vi "BatteryWarningTest_3.4V.vi"(8 "error in":errorcluster) -> (0 "error in (no error)":errorcluster, 1 "Pass/Fail":bool, 4 "Limit2":u8[](array[numeric]) format="%x", 5 "Limit1":u8[](array[numeric]) format="%x")   [LabVIEW 2009]
uses:
  Global/Global 1.vi
  <vilib>/Instr/_visa.llb/VISA Configure Serial Port (Instr).vi
panel:
  # "30"
  # "0A"
  # "0A"
  # "31"
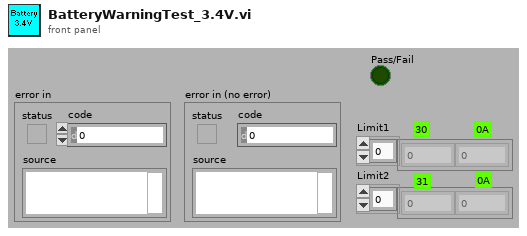
[diagram p1: front panel]
types:
  T1 = cluster{"VHEATFUSENOLOADMIN":string, "VHEATFUSELOADMAX":string, "VOVERRIDEDIODEMIN":string, "TDIFFMAX":string, "MEASFREQMAX":string, "MEASFREQMIN":string, "VOVER":string, "VMIDDLE":string, "VUNDER":string, "VNORESET":string, "VRESET":string, "WAITPING":string, "LRFID":string, "RFIDUID":string, "EXTEESIZE":string, "LCUTYPE":string, "LCUSUBTYPE":string, "TEVN":string, "BOOTVER":string, "APPVER":string, "ISLEEPMAX":string, "TSLEEP":string, "APPWAIT":string, "DBWAIT":string}
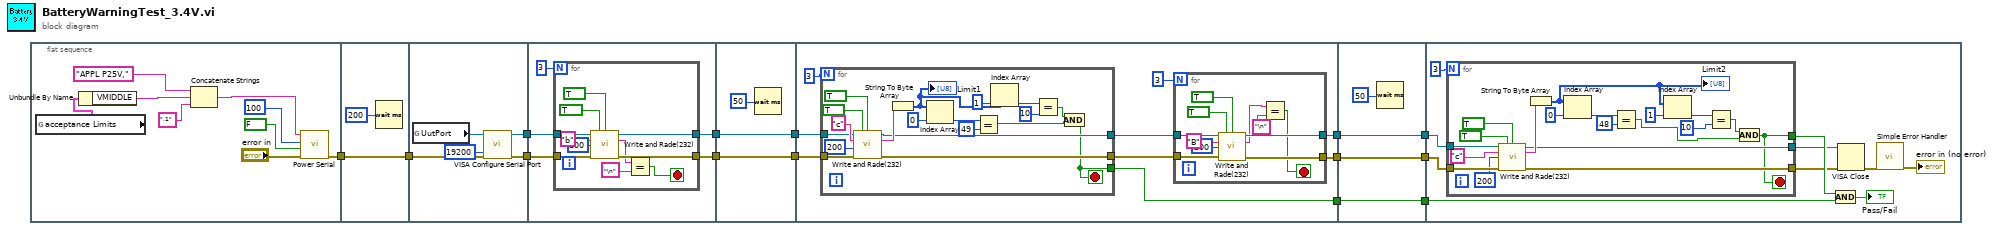
[diagram p0: block diagram]
diagram:
  n1 = flat-sequence {
    tunnel: [w20] -> w1
    tunnel: w1 -> [w25]
    tunnel: [w25] -> w2
    tunnel: [w30] -> w12
    tunnel: [w29] -> w11
    tunnel: w2 -> [w26]
    tunnel: w12 -> [w35]
    tunnel: w11 -> [w34]
    tunnel: [w33] -> w10
    tunnel: [w32] -> w8
    tunnel: w10 -> [w48]
    tunnel: [w48] -> w9
    tunnel: w8 -> [w47]
    tunnel: [w47] -> w7
    tunnel: [w58] -> w13
    tunnel: [w55] -> w6
    tunnel: [w54] -> w3
    tunnel: w7 -> [w51]
    tunnel: w9 -> [w52]
    tunnel: [w91] -> w14
    tunnel: w13 -> [w91]
    tunnel: w6 -> [w90]
    tunnel: [w90] -> w5
    tunnel: [w89] -> w4
    tunnel: w3 -> [w89]
    tunnel: w14 -> [w102]
    tunnel: w5 -> [w99]
    tunnel: w4 -> [w98]
    frame #0 {
      n2 = global read "Global 1.vi" "acceptance Limits"() -> (w19:T1)
      n3 = Unbundle By Name(w19) -> ("VMIDDLE"=w18:string)
      n4 = Concatenate Strings("APPL P25V," ("In"), w18, ",1" ("string")) -> (w15:string)
      n5 = call "Power Serial.vi"("error in (no error)"="error in", "Rd?"=FALSE, "Delay"=100, "IN"=w15) -> ("error out"=w20:errorcluster)  [unwired: 1 in, 6 out]
    }
    frame #1 {
      n6 = Wait (ms)(milliseconds to wait=u32 200) -> ()  [unwired: 1 out]
    }
    frame #2 {
      n7 = global read "Global 1.vi" "UutPort"() -> (w28:refnum<visa-resource-name>)
      n8 = call-poly "VISA Configure Serial Port"("VISA resource name"=w28, "baud rate (9600)"=u32 19200, "error in (no error)"=w26) -> ("VISA resource name out"=w29:refnum<visa-resource-name>, "error out"=w30:errorcluster)  [unwired: 3 in, 8 out]
    }
    frame #3 {
      n9 = for {
        N: 3 -> [_]
        tunnel: w35 -> [w45]
        tunnel: w34 -> [w44]
        tunnel: [w43] -> w33
        tunnel: [w42] -> w32
        stop <- w37 stop-if-true
        n10 = call "Write and Rade(232).vi"("VISA resource name in"=w44, "write"=TRUE, "read"=TRUE, "string to write"="b", "ms delay"=u32 100, "error in"=w45) -> ("VISA resource name out"=w43:refnum<visa-resource-name>, "read string"=w39:string, "error out"=w42:errorcluster)  [unwired: 2 in, 5 out]
        n11 = Equal?(x=w39, y="\n") -> (x = y?=w37:bool)
      }
    }
    frame #4 {
      n12 = Wait (ms)(milliseconds to wait=u32 50) -> ()  [unwired: 1 out]
    }
    frame #5 {
      n13 = for {
        N: 3 -> [_]
        tunnel: [w60] -> w58
        tunnel: w52 -> [w66]
        tunnel: w51 -> [w63]
        tunnel: [w62] -> w57
        tunnel: [w61] -> w56
        stop <- w60 stop-if-true
        n14 = call "Write and Rade(232).vi"("VISA resource name in"=w66, "write"=TRUE, "read"=TRUE, "string to write"="c", "ms delay"=u32 200, "error in"=w63) -> ("VISA resource name out"=w62:refnum<visa-resource-name>, "read string"=w67:string, "error out"=w61:errorcluster)  [unwired: 2 in, 5 out]
        n15 = String To Byte Array(string=w67) -> (unsigned byte array=w72:u8[])
        "Limit1" <- w72
        n16 = Index Array(array=w72, index=0) -> (element=w70:u8)
        n17 = Equal?(x=w70, y=u8 49) -> (x = y?=w77:bool)
        n18 = Index Array(array=w72, index=1) -> (element=w74:u8)
        n19 = Equal?(x=w74, y=u8 10) -> (x = y?=w76:bool)
        n20 = And(x=w76, y=w77) -> (x .and. y?=w60:bool)
      }
      n21 = for {
        N: 3 -> [_]
        tunnel: w57 -> [w87]
        tunnel: w56 -> [w84]
        tunnel: [w83] -> w55
        tunnel: [w82] -> w54
        stop <- w79 stop-if-true
        n22 = call "Write and Rade(232).vi"("VISA resource name in"=w87, "write"=TRUE, "read"=TRUE, "string to write"="B", "ms delay"=u32 200, "error in"=w84) -> ("VISA resource name out"=w83:refnum<visa-resource-name>, "read string"=w81:string, "error out"=w82:errorcluster)  [unwired: 2 in, 5 out]
        n23 = Equal?(x=w81, y="\n") -> (x = y?=w79:bool)
      }
    }
    frame #6 {
      n24 = Wait (ms)(milliseconds to wait=u32 50) -> ()  [unwired: 1 out]
    }
    frame #7 {
      n25 = for {
        N: 3 -> [_]
        tunnel: [w104] -> w100
        tunnel: w99 -> [w111]
        tunnel: w98 -> [w110]
        tunnel: [w106] -> w96
        tunnel: [w105] -> w93
        stop <- w104 stop-if-true
        n26 = call "Write and Rade(232).vi"("VISA resource name in"=w111, "write"=TRUE, "read"=TRUE, "string to write"="c", "ms delay"=u32 200, "error in"=w110) -> ("VISA resource name out"=w105:refnum<visa-resource-name>, "read string"=w107:string, "error out"=w106:errorcluster)  [unwired: 2 in, 5 out]
        n27 = String To Byte Array(string=w107) -> (unsigned byte array=w117:u8[])
        "Limit2" <- w117
        n28 = Index Array(array=w117, index=0) -> (element=w115:u8)
        n29 = Equal?(x=w115, y=u8 48) -> (x = y?=w121:bool)
        n30 = Index Array(array=w117, index=1) -> (element=w119:u8)
        n31 = Equal?(x=w119, y=u8 10) -> (x = y?=w113:bool)
        n32 = And(x=w113, y=w121) -> (x .and. y?=w104:bool)
      }
      n33 = And(x=w100, y=w102) -> (x .and. y?=→"Pass/Fail":bool)
      n34 = VISA Close(VISA resource name=w93, error in (no error)=w96) -> (error out=w95:errorcluster)
      n35 = call <vilib>:"Simple Error Handler.vi"("error in (no error)"=w95) -> ("error out"=→"error in (no error)":errorcluster)  [unwired: 1 in, 7 out]
    }
  }
